vi "Read Thread States.vi"(8 "error in (no error)":errorcluster, 11 "Framework in":refnum<class "Framework.lvclass">) -> (0 "error out":errorcluster, 1 "public thread states":T1[](array[typedef]), 2 "private thread states":T1[](array[typedef]), 3 "Framework out":refnum<class "Framework.lvclass">)   [LabVIEW 2017, in "DSF Core.lvlib" / "Framework.lvclass"]
uses:
  Framework.lvclass
  Thread/Thread State.ctl
  Framework.lvclass/Framework.ctl
  Thread Manager/Thread Manager.lvclass
  Thread/Thread.lvclass
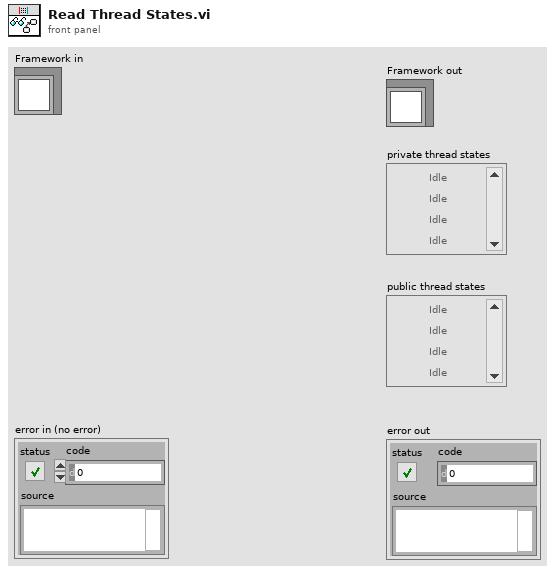
[diagram p1: front panel]
types:
  T1 = typedef "DSF Core.lvlib/Thread.lvclass/Thread State.ctl" = enum8{"Idle", "Running", "Error", "Shut Down"}
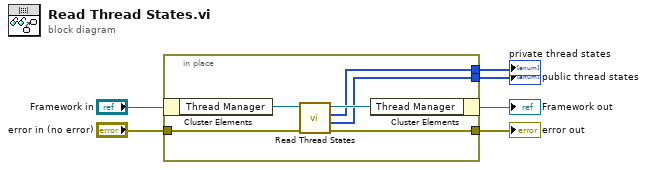
[diagram p0: block diagram]
diagram:
  n1 = in-place {
    in-place-border: "error in (no error)" -> [w10]
    in-place-border: [w9] -> w4
    in-place-border: [w7] -> w5
    in-place-border: [w8] -> w6
    n2 = in-place-cluster #1("Framework in") -> ("Thread Manager"=w12:refnum<class "Thread Manager.lvclass">)
    n3 = call "Read Thread States.vi"("error in (no error)"=w10, "Thread Manager in"=w12) -> ("error out"=w9:errorcluster, "public thread states"=w7:T1[], "private thread states"=w8:T1[], "Thread Manager out"=w11:refnum<class "Thread Manager.lvclass">)  [unwired: 6 in]
    n4 = in-place-cluster #1("Thread Manager"=w11) -> (→"Framework out":refnum<class "Framework.lvclass">)
  }
  "private thread states" <- w6
  "public thread states" <- w5
  "error out" <- w4
